vi "Thorlabs_SC10_Serial.vi"() -> ()   [LabVIEW 2022 SP3]
uses:
  Program Files/National Instruments/LabVIEW 2022/examples/Instrument IO/Serial/support/Serial - Settings.ctl
  <vilib>/Instr/_visa.llb/VISA Configure Serial Port (Instr).vi
panel:
  out "Open?":bool
  out "error out":errorcluster
  in  "error in (no error)":errorcluster
  in  "stop":bool
  in  "Open/close":bool
  in  "VISA resource name":refnum<visa-resource-name>="COM1"
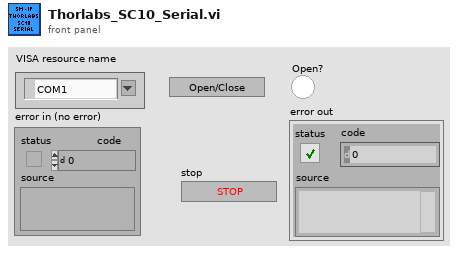
[diagram p1: front panel]
types:
  T1 = typedef "Serial - Settings.ctl" = cluster{"baud rate":u32, "data bits":u16, "parity":enum16{"None", "Odd", "Even", "Mark", "Space"}, "stop bits":u16, "flow control":u16}
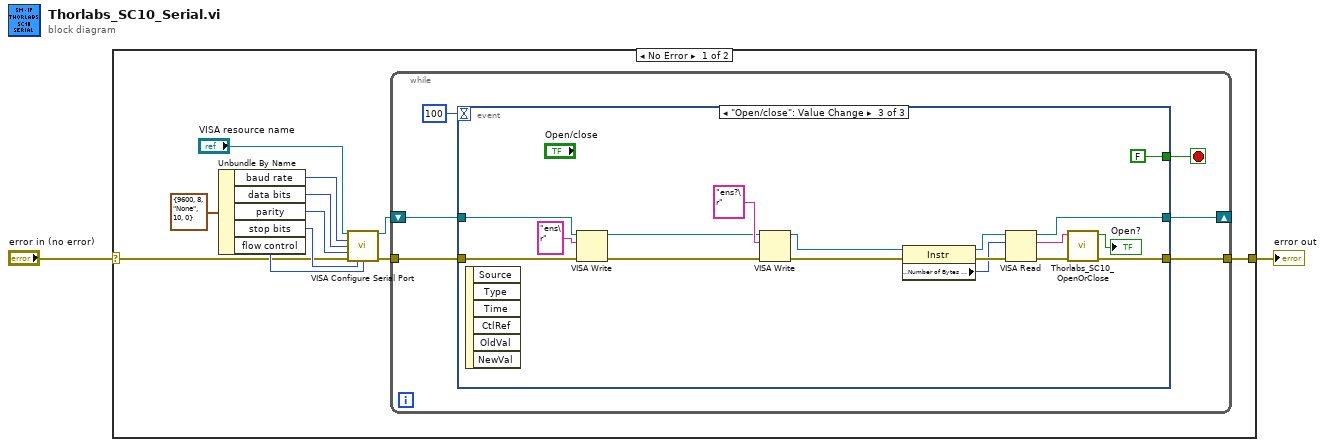
[diagram p0: block diagram]
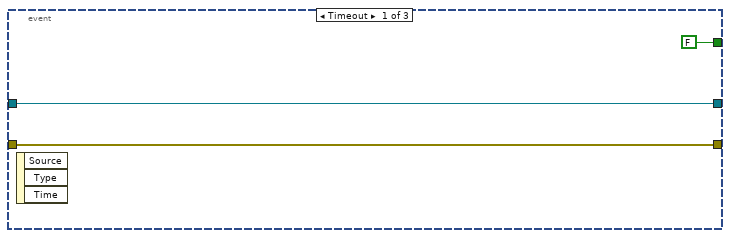
[diagram p2: hidden frame]
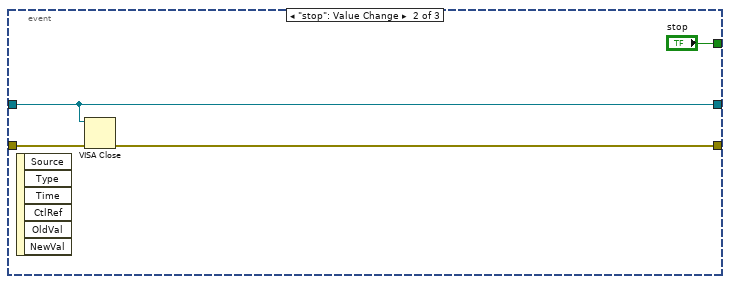
[diagram p3: hidden frame]
diagram:
  n1 = case shown="No Error" "error in (no error)" {
    selector: "error in (no error)" -> [w3 w44]
    tunnel: [w4 w44] -> w2
    frame No Error {
      n2 = Unbundle By Name(T1 {"baud rate"=9600, "data bits"=8, "parity"=enum."None", "stop bits"=10, "flow control"=0} ("Serial Settings")) -> ("baud rate"=w9:u32, "data bits"=w10:u16, "parity"=w11:enum16{"None", "Odd", "Even", "Mark", "Space"}, "stop bits"=w12:u16, "flow control"=w13:u16)
      n3 = call-poly "VISA Configure Serial Port"("VISA resource name"="VISA resource name", "baud rate (9600)"=w9, "data bits (8)"=w10, "parity (0:none)"=w11, "error in (no error)"=w3, "stop bits (10: 1 bit)"=w12, "flow control (0:none)"=w13) -> ("VISA resource name out"=w6:refnum<visa-resource-name>, "error out"=w5:errorcluster)  [unwired: 2 in, 5 out]
      n4 = while {
        tunnel: w5 -> [w18]
        shift-right: [w14] -> _
        shift-left: w6 -> [w17]
        tunnel: [w15] -> w4
        stop <- w16 stop-if-true
        n5 = event shown="[2] \"Open/close\": Value Change" {
          selector: _ -> [_ _ _]
          dyn-events: _ -> [_ _ _]
          timeout: 100 -> [_ _ _]
          tunnel: w18 -> [w20 w25 w42]
          tunnel: w17 -> [w21 w23 w41]
          tunnel: [w21 w23 w33] -> w14
          tunnel: [FALSE ("stop") "stop" FALSE ("stop")] -> w16
          tunnel: [w20 w24 w31] -> w15
          event Timeout {
            n6 = event-data() -> ()  [unwired: 1 in, 3 out]
          }
          event "stop": Value Change {
            n7 = event-data() -> ()  [unwired: 1 in, 6 out]
            n8 = VISA Close(VISA resource name=w23, error in (no error)=w25) -> (error out=w24:errorcluster)
          }
          event "Open/close": Value Change {
            n9 = event-data() -> ()  [unwired: 1 in, 6 out]
            n10 = VISA Write(VISA resource name=w41, write buffer="ens\r" ("Command"), error in (no error)=w42) -> (VISA resource name out=w35:refnum<visa-resource-name>, error out=w34:errorcluster)  [unwired: 1 out]
            n11 = VISA Write(VISA resource name=w35, write buffer="ens?\r" ("Command"), error in (no error)=w34) -> (VISA resource name out=w28:refnum<visa-resource-name>, error out=w27:errorcluster)  [unwired: 1 out]
            n12 = property class="Instr"(reference=w28, error in=w27) -> (reference out=w38:refnum<visa-resource-name>, error out=w37:errorcluster, "Serial Settings:Number of Bytes at Serial Port"=w36:u32)
            n13 = VISA Read(VISA resource name=w38, byte count=w36, error in (no error)=w37) -> (VISA resource name out=w33:refnum<visa-resource-name>, read buffer=w32:string, error out=w30:errorcluster)  [unwired: 1 out]
            n14 = call "Thorlabs_SC10_OpenOrClose.vi"("error in (no error)"=w30, "Input string"=w32) -> ("error out"=w31:errorcluster, "Open?"=→"Open?":bool)  [unwired: 8 in]
          }
        }
      }
    }
    frame Error {
    }
  }
  "error out" <- w2
